vi "1D STR Array_DeleteCellsWithSpecifiedValue.vi"(1 "CellValueToBeDeleted":string, 2 "1D STR Array.IN":string[](array[string])=["", ""]) -> (6 "1D STR Array.OUT":string[](array[string]))   [LabVIEW 2024]
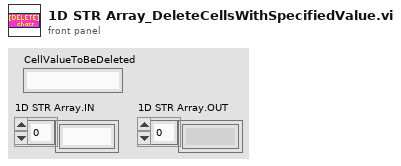
[diagram p1: front panel]
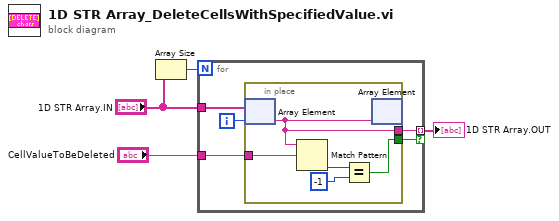
[diagram p0: block diagram]
diagram:
  n1 = Array Size(array="1D STR Array.IN") -> (size(s)=w4:i32)
  n2 = for {
    N: w4 -> [_]
    tunnel: "1D STR Array.IN" -> [w9]
    tunnel: [w7] -> w2 mode=indexing if=w5
    tunnel: "CellValueToBeDeleted" -> [w6]
    i -> [w8]
    n3 = in-place {
      in-place-border: [w13] -> w7
      in-place-border: w6 -> [w12]
      in-place-border: [w14] -> w5
      n4 = in-place-array #1(w9, w8) -> (w13:string)
      n5 = Match Pattern(string=w13, regular expression=w12) -> (offset past match=w11:i32)  [unwired: 1 in, 3 out]
      n6 = Equal?(x=w11, y=-1) -> (x = y?=w14:bool)
      n7 = in-place-array #1(w13) -> ()  [unwired: 2 out]
    }
  }
  "1D STR Array.OUT" <- w2
